vi "Write_Read_VISA.vi"(8 "error in (no error)":errorcluster {"code" format="%.0x"}, 9 "Return Byte":u32=4, 10 "write buffer":string, 11 "VISA session":refnum<visa-resource-name>) -> (0 "error out":errorcluster {"code" format="%.0x"}, 2 "read buffer":string, 3 "dup VISA session":refnum<visa-resource-name>)   [LabVIEW 2018]
doc: "This VI displays the results of the selected continual display measurement."
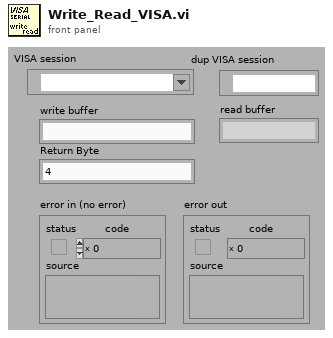
[diagram p1: front panel]
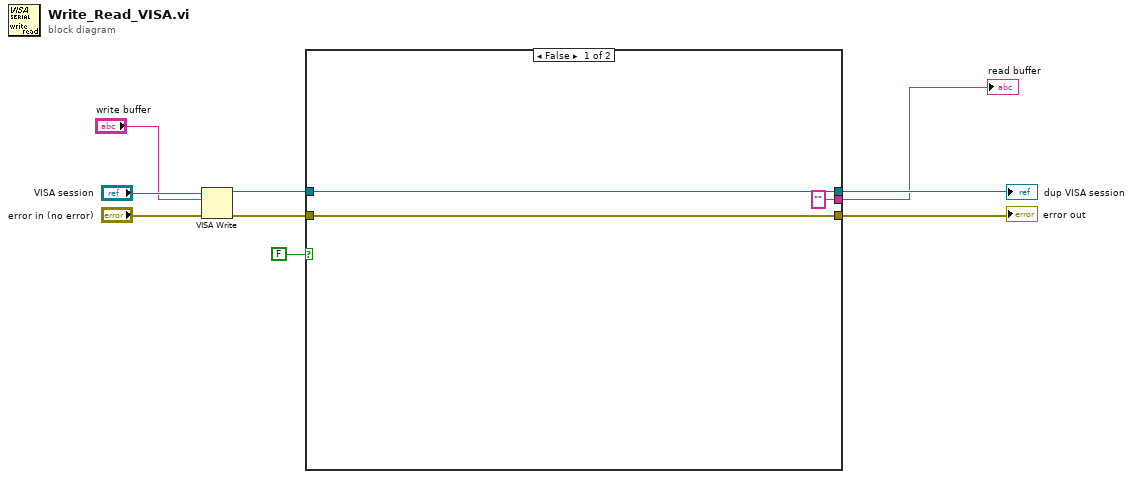
[diagram p0: block diagram]
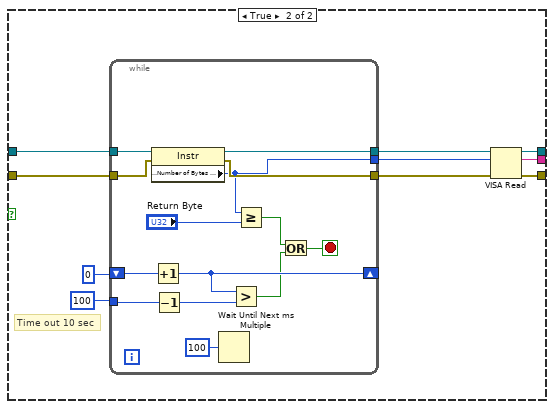
[diagram p2: hidden frame]
diagram:
  n1 = VISA Write(VISA resource name="VISA session", write buffer="write buffer", error in (no error)="error in (no error)") -> (VISA resource name out=w5:refnum<visa-resource-name>, error out=w4:errorcluster)  [unwired: 1 out]
  n2 = case shown="False" FALSE {
    tunnel: [w11 w22] -> w7
    tunnel: [w12 w21] -> w6
    tunnel: w5 -> [w12 w20]
    tunnel: w4 -> [w11 w19]
    tunnel: ["" ("read buffer") w15] -> w2
    frame False {
    }
    frame True {
      # "Time out 10 sec"
      n3 = while {
        tunnel: w20 -> [w36]
        tunnel: w19 -> [w35]
        tunnel: [w34] -> w18
        tunnel: [w33] -> w17
        tunnel: [w32] -> w16
        shift-right: [w30] -> _
        shift-left: u32 0 ("millisecond multiple") -> [w25]
        tunnel: u32 100 ("millisecond multiple") -> [w24]
        stop <- w27 stop-if-true
        n4 = property class="Instr"(reference=w36, error in=w35) -> (reference out=w34:refnum<visa-resource-name>, error out=w33:errorcluster, "Serial Settings:Number of Bytes at Serial Port"=w32:u32)
        n5 = Increment(x=w25) -> (x+1=w30:u32)
        n6 = Decrement(x=w24) -> (x-1=w23:u32)
        n7 = Wait Until Next ms Multiple(millisecond multiple=u32 100) -> ()  [unwired: 1 out]
        n8 = Greater?(x=w30, y=w23) -> (0:w28:bool)
        n9 = Greater Or Equal?(x=w32, y="Return Byte") -> (x >= y?=w29:bool)
        n10 = Or(x=w29, y=w28) -> (x .or. y?=w27:bool)
      }
      n11 = VISA Read(VISA resource name=w18, byte count=w16, error in (no error)=w17) -> (VISA resource name out=w21:refnum<visa-resource-name>, read buffer=w15:string, error out=w22:errorcluster)  [unwired: 1 out]
    }
  }
  "error out" <- w7
  "dup VISA session" <- w6
  "read buffer" <- w2
